vi "Elevator Reach Height.vi"(7 "PID gains":T1={"proportional gain (Kc)"=1.0, "integral time (Ti, min)"=0.01, "derivative time (Td, min)"=0.0} {"derivative time (Td, min)" format="%.3f"; "integral time (Ti, min)" format="%.3f"; "proportional gain (Kc)" format="%.3f"}, 8 "Elevator Tolerance":dbl, 9 "Reset Encoders":bool, 10 "output range":cluster{"output high":dbl, "output low":dbl}={"output high"=100.0, "output low"=-100.0} {"output low" format="%.2f"; "output high" format="%.2f"}, 11 "Reach Height":dbl) -> (1 "Distance":dbl, 2 "Finished":bool, 3 "Output":dbl)   [LabVIEW 2017]
uses:
  Common Code/PID Gains.ctl
  <vilib>/addons/control/pid/pid.llb/PID (DBL).vi
  <vilib>/addons/control/pid/NI_PID_pid.lvlib
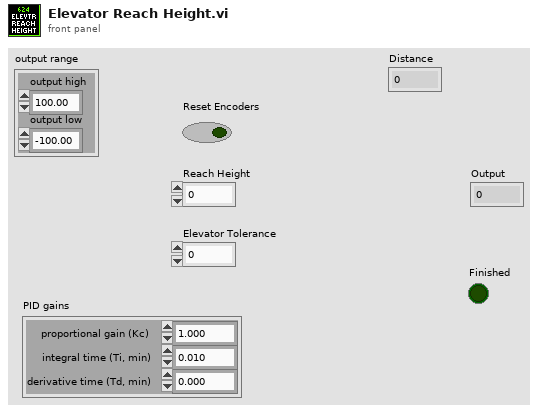
[diagram p1: front panel]
types:
  T1 = typedef "PID Gains.ctl" = cluster{"proportional gain (Kc)":dbl, "integral time (Ti, min)":dbl, "derivative time (Td, min)":dbl}
  T2 = typedef "Encoder Values.ctl" = cluster{"Distance":dbl, "Speed":dbl, "Tick":dbl}
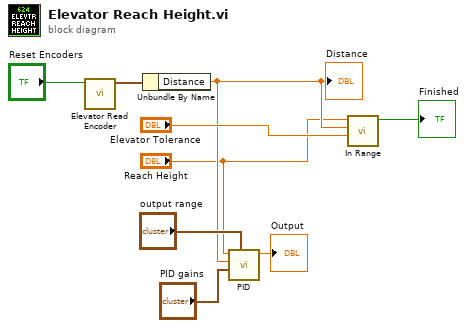
[diagram p0: block diagram]
diagram:
  n1 = call "Elevator Read Encoder.vi"("Reset Encoders"="Reset Encoders") -> ("Encoder Values"=w7:T2)  [unwired: 10 in]
  n2 = Unbundle By Name(w7) -> ("Distance"=w2:dbl)
  "Distance" <- w2
  n3 = call-poly <vilib>:"PID.vi"("output range"="output range", "PID gains"="PID gains", "process variable"=w2, "setpoint"="Reach Height") -> ("output"=→"Output":dbl)  [unwired: 6 in, 1 out]
  n4 = call "In Range.vi"("Tolerance"="Elevator Tolerance", "Encoder Height"=w2, "Height"="Reach Height") -> ("In Range"=→"Finished":bool)  [unwired: 8 in]
